vi "data array to formatted string.vi"(1 "data array":sgl[](array[numeric])=[0.0, 0.0, 0.0, 0.0]) -> (0 "formatted string":string)   [LabVIEW 2016]
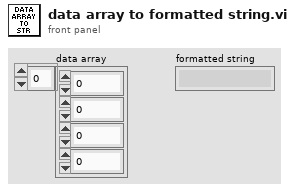
[diagram p1: front panel]
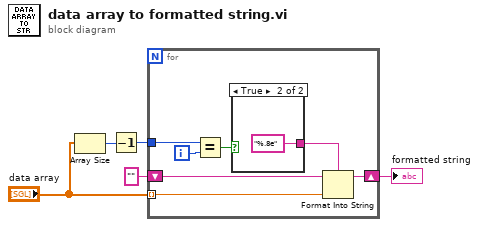
[diagram p0: block diagram]
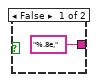
[diagram p2: hidden frame]
diagram:
  n1 = Array Size(array="data array") -> (size(s)=w3:i32)
  n2 = Decrement(x=w3) -> (x-1=w2:i32)
  n3 = for {
    tunnel: "data array" -> [w11] mode=indexing
    shift-right: [w6] -> w1
    shift-left: "" -> [w12]
    tunnel: w2 -> [w9]
    i -> [w8]
    n4 = Equal?(x=w9, y=w8) -> (x = y?=w7:bool)
    n5 = case shown="True" w7 {
      tunnel: ["%.8e," ("format string") "%.8e" ("format string")] -> w10
      frame False {
      }
      frame True {
      }
    }
    n6 = Format Into String(format string=w10, initial string=w12, w11) -> (resulting string=w6:string)  [unwired: 1 in, 1 out]
  }
  "formatted string" <- w1
